vi "Calc Dark Array.vi"(8 "error in (no error)":errorcluster, 10 "file path (dialog if empty)":path=path "C:/Users/dhstuart/Dropbox/CLTC/avantesSpectrometer/Cal Files/Dark Model Parameters.csv", 11 "intTime":dbl format="%#_13g") -> (0 "error out":errorcluster, 3 "Dark Array":dbl[](array[numeric]))   [LabVIEW 2013]
uses:
  <vilib>/Analysis/1siggen.llb/Ramp Pattern by Delta.vi
  <vilib>/Utility/file.llb/Read From Spreadsheet File (DBL).vi
  <vilib>/express/express arith-compare/Formula/XNode/ExpressFormulaBlockNode.xnode
  <vilib>/Analysis/NI_AALBase.lvlib
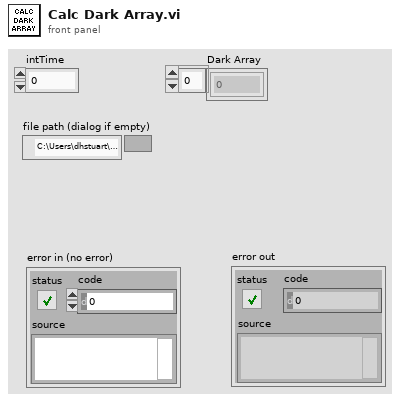
[diagram p1: front panel]
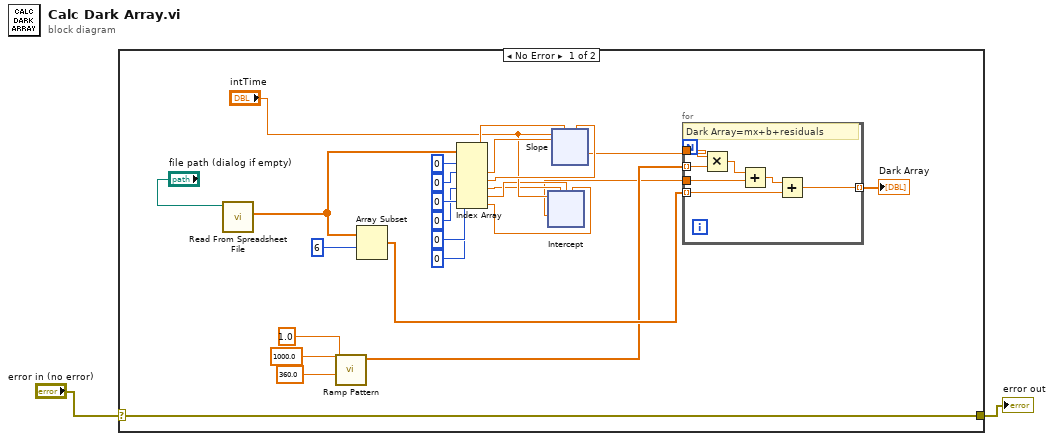
[diagram p0: block diagram]
diagram:
  n1 = case shown="No Error" "error in (no error)" {
    selector: "error in (no error)" -> [w3 w63]
    tunnel: [w3 w63] -> w1
    frame No Error {
      n2 = call-poly <vilib>:"Read From Spreadsheet File.vi"("file path (dialog if empty)"="file path (dialog if empty)") -> ("first row"=w25:dbl[])  [unwired: 6 in, 4 out]
      n3 = call-poly <vilib>:"Ramp Pattern.vi"("start"=360.0, "end"=1000.0, "delta"=1.0) -> ("Ramp Pattern"=w7:dbl[])  [unwired: 6 in, 2 out]
      n4 = Array Subset(array=w25, index=6) -> (w11:dbl[])  [unwired: 1 in]
      n5 = Index Array(array=w25, index #1=0 ("index"), index #2=0 ("index"), index #3=0 ("index"), index #4=0 ("index"), index #5=0 ("index"), index #6=0 ("index")) -> (element #1=w18:dbl, element #2=w17:dbl, element #3=w16:dbl, element #4=w12:dbl, element #5=w13:dbl, element #6=w14:dbl)
      n6 = xnode "Intercept"("intTime"="intTime", "a"=w12, "b"=w13, "c"=w14) -> ("Result"=w5:dbl)  [unwired: 1 in, 1 out]
      n7 = xnode "Slope"("intTime"="intTime", "a"=w18, "b"=w17, "c"=w16) -> ("Result"=w6:dbl)  [unwired: 1 in, 1 out]
      n8 = for {
        tunnel: w11 -> [w29] mode=indexing
        tunnel: w7 -> [w33] mode=indexing
        tunnel: w6 -> [w34]
        tunnel: w5 -> [w31]
        tunnel: [w28] -> w4 mode=indexing
        # "Dark Array=mx+b+residuals"
        n9 = Multiply(x=w34, y=w33) -> (x*y=w32:dbl)
        n10 = Add(x=w32, y=w31) -> (x+y=w30:dbl)
        n11 = Add(x=w30, y=w29) -> (x+y=w28:dbl)
      }
      "Dark Array" <- w4
    }
    frame Error {
    }
  }
  "error out" <- w1
